vi "Configure Internal Switch.vi"(0 "VISA resource name":refnum<visa-resource-name>, 5 "Internal Switch Number (1)":i32=1 min=1 max=100, 7 "Output Type (0: Alarm)":u16(ring) items=["Alarm", "Manual"], 9 "Internal Switch Operation (1: Or)":u16(ring)=1 items=["And", "Or"], 11 "error in (no error)":errorcluster) -> (4 "VISA resource name out":refnum<visa-resource-name>, 6 "Internal Switch Number":i32, 15 "error out":errorcluster)   [LabVIEW 2020, in "Yokogawa GX Series.lvlib"]
doc: "Sets the internal switch operation.\n\nCommand: SSwitch"
uses:
  <instrlib>/Yokogawa GX Series/Yokogawa GX Series.lvlib
panel:
  in  "Action When Power On (0: Last)":u16(ring) items=["Last", "On", "Off"]
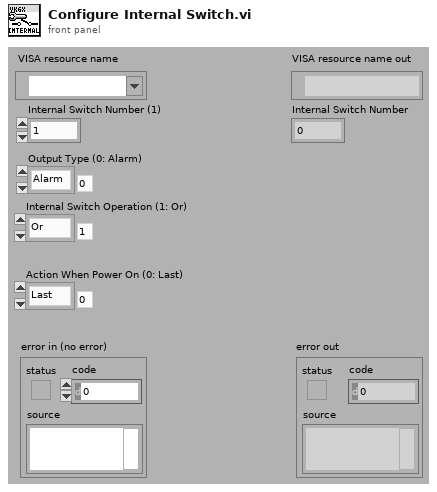
[diagram p1: front panel]
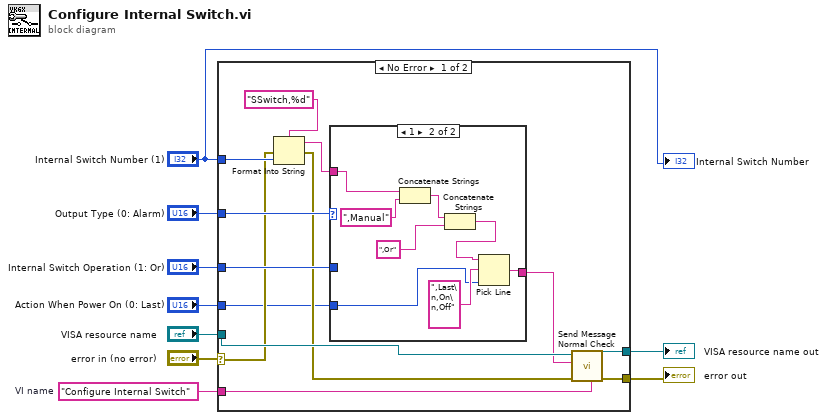
[diagram p0: block diagram]
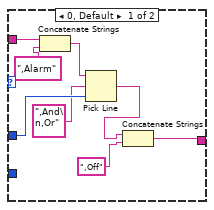
[diagram p2: hidden frame]
diagram:
  w9 = "Configure Internal Switch"  # VI name
  n1 = case shown="No Error" "error in (no error)" {
    selector: "error in (no error)" -> [w11 w39]
    tunnel: w9 -> [w22 _]
    tunnel: [w21 w40] -> w8
    tunnel: [w20 w39] -> w7
    tunnel: "VISA resource name" -> [w19 w40]
    tunnel: "Output Type (0: Alarm)" -> [w17 _]
    tunnel: "Internal Switch Operation (1: Or)" -> [w16 _]
    tunnel: "Internal Switch Number (1)" -> [w12 _]
    tunnel: "Action When Power On (0: Last)" -> [w10 _]
    frame No Error {
      n2 = Format Into String(format string="SSwitch,%d", error in=w11, w12) -> (resulting string=w15:string, error out=w13:errorcluster)  [unwired: 1 in]
      n3 = case shown="1" w17 {
        tunnel: w16 -> [w27 _]
        tunnel: w15 -> [w30 w37]
        tunnel: [w23 w34] -> w14
        tunnel: w10 -> [_ w35]
        frame 0, Default {
          n4 = Concatenate Strings(w30, ",Alarm") -> (w28:string)
          n5 = Pick Line(string ("")=w28, multi-line string=",And\n,Or", line index=w27) -> (output string=w25:string)
          n6 = Concatenate Strings(w25, ",Off") -> (w23:string)
        }
        frame 1 {
          n7 = Concatenate Strings(w37, ",Manual") -> (w33:string)
          n8 = Concatenate Strings(w33, ",Or") -> (w31:string)
          n9 = Pick Line(string ("")=w31, multi-line string=",Last\n,On\n,Off", line index=w35) -> (output string=w34:string)
        }
      }
      n10 = call <instrlib>:"Send Message Normal Check.vi"("Source (\"\")"=w22, "error in (no error)"=w13, "Send Message (\"\")"=w14, "VISA resource name"=w19) -> ("error out"=w20:errorcluster, "VISA resource name out"=w21:refnum<visa-resource-name>)  [unwired: 2 in, 4 out]
    }
    frame Error {
    }
  }
  "error out" <- w7
  "VISA resource name out" <- w8
  "Internal Switch Number" <- "Internal Switch Number (1)"
